vi "FRC Color Processing Example.vi"(8 "Image In":T1) -> ()   [LabVIEW 2015]
uses:
  <vilib>/vision/NI_Vision_Development_Module.lvlib
  Vision Support Code/Camera Types.ctl
  <vilib>/Rock Robotics/WPI/Camera/WPI_CameraSettings Read MJPG.ctl
  <vilib>/Rock Robotics/WPI/Camera/WPI_CameraImageSize.ctl
  <vilib>/vision/Image Controls.llb/IMAQ Image.ctl
panel:
  in  "Std Devs for Calibration":cluster{"H":dbl, "S":dbl, "V":dbl}={"H"=4.0, "S"=6.0, "V"=6.0}
  out "Highest Avg Score":dbl format="%#_3g"
  in  "Min Score Threshold":i32=70
  in  "Emphasize Limit Tests":bool=TRUE
  in  "Camera Type":T2=enum."MS HD3000 square"
  in  "image files":string[](array[string])
  in  "Aspect Ratio Fudge Factor":dbl=1.0
  out "Detected Targets":T3(array[cluster]) {"Normalized Rect"."Numeric 5" format="%#_2g"; "Normalized Rect"."Numeric 3" format="%#_2g"; "Normalized Rect"."Numeric 2" format="%#_2g"; "Normalized Rect"."Numeric" format="%#_2g"}
  in  "Annotation Limit":dbl=75.0
  in  "Source":enum32{"Files", "Camera"}(tab)
  in  "Images":i32(listbox)
  in  "Folder Location":path=path "C:/Program Files (x86)/National Instruments/LabVIEW 2015/examples/FRC/roboRIO/Vision/2016 Vision Example/Sample Images/Real Tower"
  in  "Camera Settings":T4={"fps"=20, "compression"=30, "Image Size"=enum."320x240"}
  in  "Camera Address":string="USB 1"
  in  "Annotate":bool=TRUE
  out "Sorted Particle Scores":T6(array[cluster]) {"Moment Factor" format="%#_3g"; "Aspect Ratio" format="%#_3g"; "Area to CH" format="%#_3g"; "X" format="%#_3g"; "Y" format="%#_3g"}
  out "Qualified Particles":i32
  in  "LED Color":T7={"Hue"={110.52399131877658, 148.6727294921875}, "Sat"={34.78571428571429, 255.0}, "Val"={91.07142857142858, 255.0}} {"Hue" scale=0.0..255.0 scale format="%#_3g"}
  out "Masked":T1(plugin-control)
  out "Original Image":T1(plugin-control)
  # "Instructions:\nUse Source to select image files from a directory, or use a USB or IP camera connected to your laptop.\nUse LED Color to threshold and build particles. Adjust HSV values to improve masking.\nClick and draw a line in Original Image to auto-calibrate to the LED color. You may need to widen Sat and Val.\nAnnotations draw a rectangle around \"good\" particles with scores from top to bottom."
  # "Density Profile"
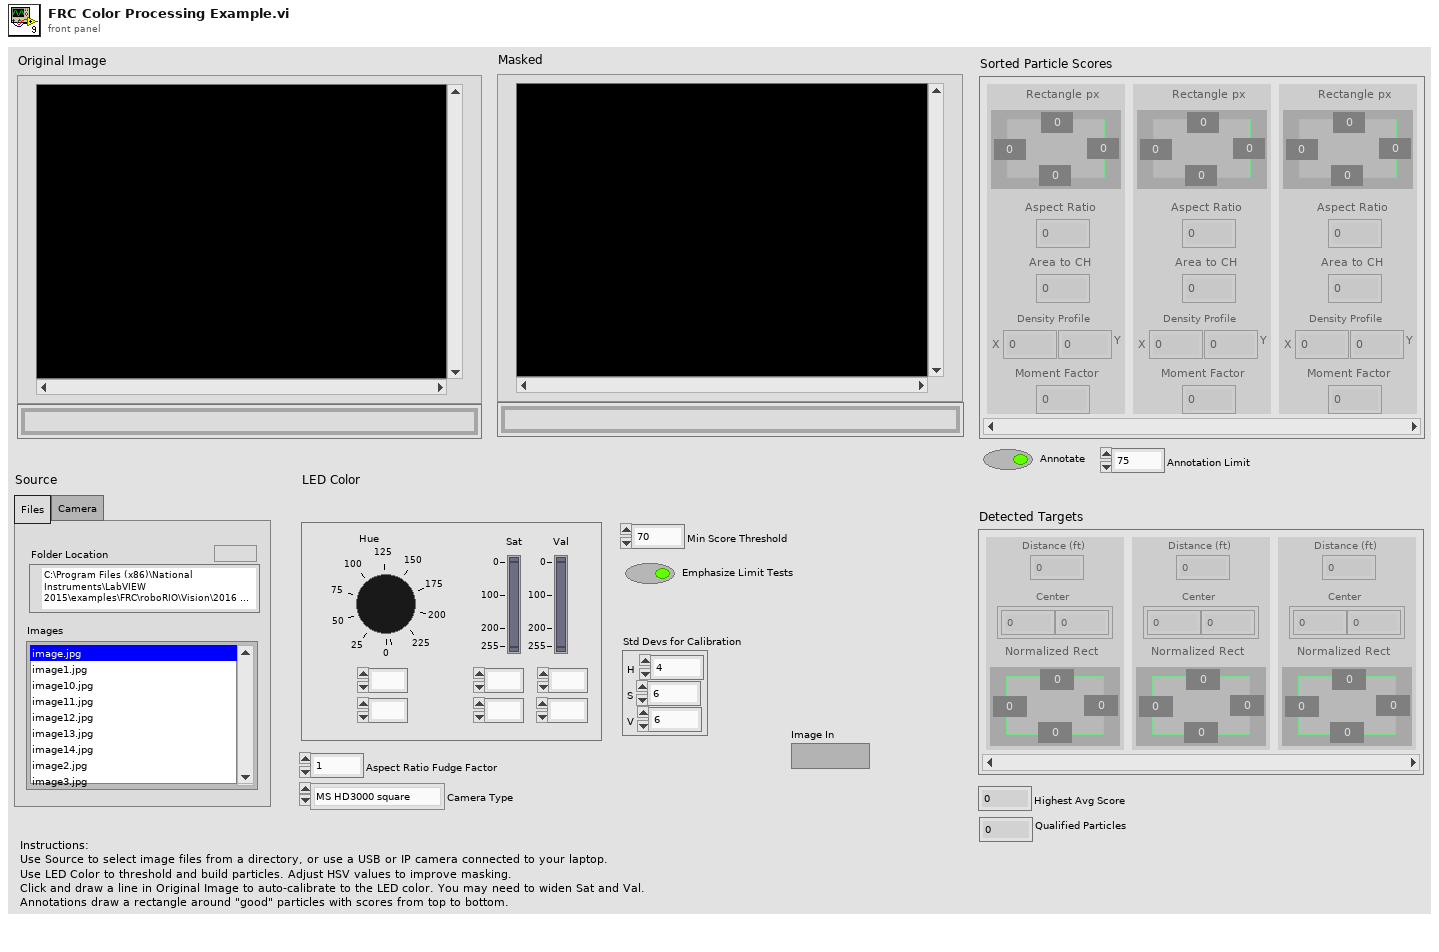
[diagram p1: front panel]
types:
  T1 = typedef "IMAQ Image.ctl" = refnum<image>
  T2 = typedef "Camera Types.ctl" = enum16{"206", "1011", "1013", "MS HD3000 square", "MS HD3000 640x480"}
  T3 = cluster{"Distance (ft)":dbl, "Center":cluster{dbl, dbl}, "Normalized Rect":cluster{"Numeric":dbl, "Numeric 2":dbl, "Numeric 3":dbl, "Numeric 5":dbl}}[]
  T4 = typedef "WPI_CameraSettings Read MJPG.ctl" = cluster{"fps":i32, "compression":i32, "Image Size":T5}
  T5 = typedef "WPI_CameraImageSize.ctl" = enum16{"640x480", "320x240", "160x120", "Custom"}
  T6 = cluster{"Rectangle px":cluster{"Numeric":dbl, "Numeric 2":dbl, "Numeric 3":dbl, "Numeric 5":dbl}, "Aspect Ratio":dbl, "Area to CH":dbl, "X":dbl, "Y":dbl, "Moment Factor":dbl}[]
  T7 = cluster{"Hue":cluster{dbl, dbl}, "Sat":cluster{dbl, dbl}, "Val":cluster{dbl, dbl}}
  T8 = typedef "Particle Parameters" = i32
  T9 = typedef "Image Type" = u32
  T10 = cluster{cluster{dbl, dbl}, cluster{dbl, dbl}, cluster{dbl, dbl}}
  T11 = cluster{"Bounding box":cluster{"left":dbl, "top":dbl, "right":dbl, "bottom":dbl}, "Aspect Ratio":dbl, "Area to CH":dbl, "X Mask":dbl, "Y Mask":dbl, "Moment":dbl}[]
  T12 = cluster{"Rectangle":cluster{"Numeric":dbl, "Numeric 2":dbl, "Numeric 3":dbl, "Numeric 5":dbl}, "L":dbl, "Area to CH":dbl, "X":dbl, "Y":dbl, "Moment Factor":dbl}[]
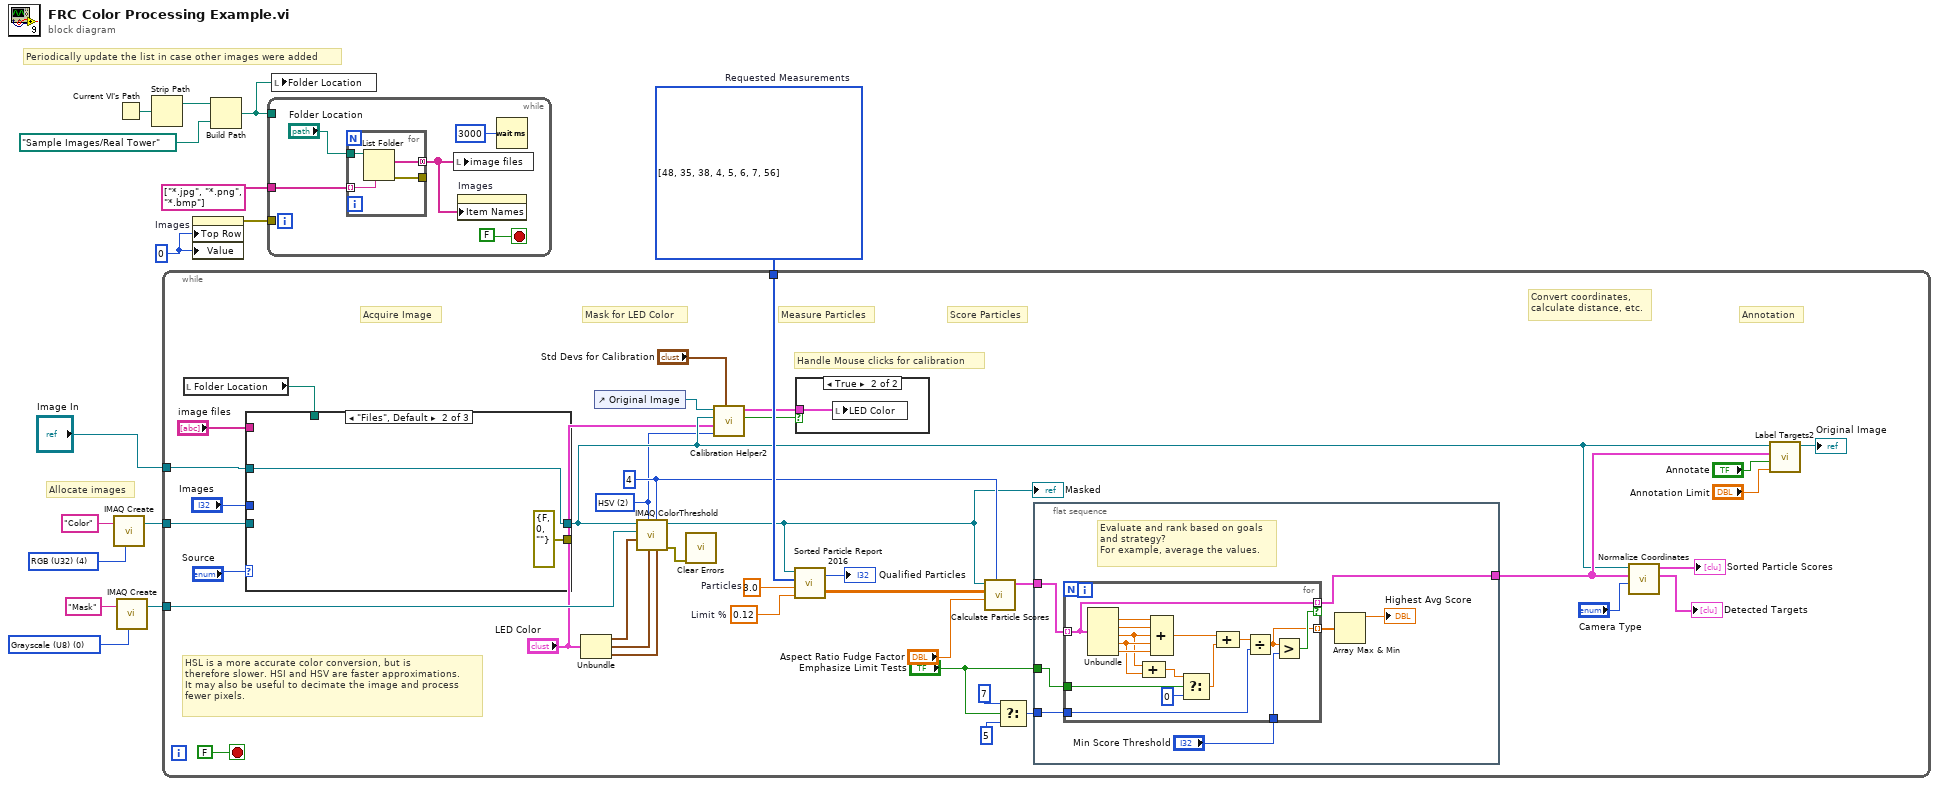
[diagram p0: block diagram]
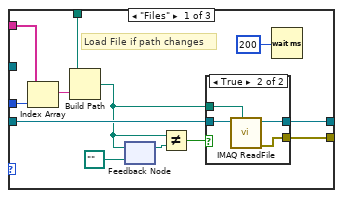
[diagram p3: hidden frame]
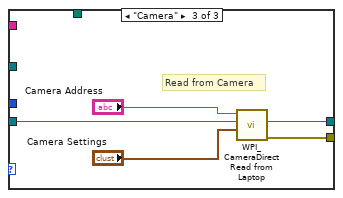
[diagram p5: hidden frame]
diagram:
  w3 = u32 0 ("milliseconds to wait")
  w9 = T8[] [48, 35, 38, 4, 5, 6, 7, 56] items=["Center of Mass X", "Center of Mass Y", "First Pixel X", "First Pixel Y", "Bounding Rect Left", "Bounding Rect Top", "Bounding Rect Right", "Bounding Rect Bottom", "Max Feret Diameter Start X", "Max Feret Diameter Start Y", "Max Feret Diameter End X", "Max Feret Diameter End Y", "Max Horiz. Segment Length Left", "Max Horiz. Segment Length Right", "Max Horiz. Segment Length Row", "-", "Bounding Rect Width", "Bounding Rect Height", "Bounding Rect Diagonal", "Perimeter", "Convex Hull Perimeter", "Holes' Perimeter", "Max Feret Diameter", "Equivalent Ellipse Major Axis", "Equivalent Ellipse Minor Axis", "Equivalent Ellipse Minor Axis (Feret)", "Equivalent Rect Long Side", "Equivalent Rect Short Side", "Equivalent Rect Diagonal", "Equivalent Rect Short Side (Feret)", "Average Horiz. Segment Length", "Average Vert. Segment Length", "Hydraulic Radius", "Waddel Disk Diameter", "-", "Area", "Holes' Area", "Particle & Holes' Area", "Convex Hull Area", "Image Area", "-", "Number of Holes", "Number of Horiz. Segments", "Number of Vert. Segments", "-", "Orientation", "Max Feret Diameter Orientation", "-", "% Area/Image Area", "% Area/(Particle & Holes' Area)", "Ratio of Equivalent Ellipse Axes", "Ratio of Equivalent Rect Sides", "-", "Elongation Factor", "Compactness Factor", "Heywood Circularity Factor", "Type Factor", "-", "Sum X", "Sum Y", "Sum XX", "Sum XY", "Sum YY", "Sum XXX", "Sum XXY", "Sum XYY", "Sum YYY", "-", "Moment of Inertia XX", "Moment of Inertia XY", "Moment of Inertia YY", "Moment of Inertia XXX", "Moment of Inertia XXY", "Moment of Inertia XYY", "Moment of Inertia YYY", "Norm. Moment of Inertia XX", "Norm. Moment of Inertia XY", "Norm. Moment of Inertia YY", "Norm. Moment of Inertia XXX", "Norm. Moment of Inertia XXY", "Norm. Moment of Inertia XYY", "Norm. Moment of Inertia YYY", "Hu Moment 1", "Hu Moment 2", "Hu Moment 3", "Hu Moment 4", "Hu Moment 5", "Hu Moment 6", "Hu Moment 7"]  # Requested Measurements
  w12 = T9 0 items=["Grayscale (U8)", "Grayscale (I16)", "Grayscale (SGL)", "Complex (CSG)", "RGB (U32)", "HSL (U32)", "RGB (U64)", "Grayscale (U16)"] ("Image Type")
  w14 = T9 4 items=["Grayscale (U8)", "Grayscale (I16)", "Grayscale (SGL)", "Complex (CSG)", "RGB (U32)", "HSL (U32)", "RGB (U64)", "Grayscale (U16)"] ("Image Type")
  # "Periodically update the list in case other images were added"
  # "Allocate images"
  n1 = call "IMAQ Create"("Image Name"="Color", "Image Type"=w14) -> ("New Image"=w13:T1)  [unwired: 2 in, 2 out]
  n2 = Current VI's Path() -> (path=w8:path)
  n3 = call "IMAQ Create"("Image Name"="Mask", "Image Type"=w12) -> ("New Image"=w10:T1)  [unwired: 2 in, 2 out]
  n4 = Strip Path(path=w8) -> (stripped path=w6:path)  [unwired: 1 out]
  n5 = while {
    tunnel: w13 -> [w53]
    tunnel: w10 -> [w51]
    tunnel: w9 -> [w47]
    tunnel: "Image In" -> [w16]
    stop <- FALSE stop-if-true
    w39 = 4 ("Replace Value")
    w43 = 0.12  # Limit %
    w46 = 3.0  # Particles
    w21 = u16 2 items=["RGB", "HSL", "HSV", "HSI"] ("Color Mode")
    # "Handle Mouse clicks for calibration"
    # "Measure Particles"
    # "Convert coordinates,\ncalculate distance, etc."
    # "Annotation"
    # "Score Particles"
    # "Mask for LED Color"
    # "Acquire Image"
    # "HSL is a more accurate color conversion, but is\ntherefore slower. HSI and HSV are faster approximations.\nIt may also be useful to decimate the image and process\nfewer pixels."
    n6 = local read "Folder Location"() -> (w18:path)
    n7 = case shown="Default, \"Robot\"" "Source" {
      tunnel: [w89 errorcluster {"status"=FALSE, "code"=0, "source"=""} ("error out") w102] -> _
      tunnel: [w90 w97 w101] -> w24
      tunnel: w53 -> [w88 _ w100]
      tunnel: "image files" -> [w80 _ _]
      tunnel: "Images" -> [w87 _ _]
      tunnel: w18 -> [w85 _ _]
      tunnel: w16 -> [_ w97 _]
      frame "Files" {
        # "Load File if path changes"
        n8 = Index Array(array=w80, index=w87) -> (element=w86:string)
        n9 = Build Path(base path=w85, name or relative path=w86) -> (appended path=w81:path)
        n10 = feedback-in #1(w81) -> ()
        n11 = feedback #1(path "" ("appended path")) -> (w83:path)
        n12 = Not Equal?(x=w81, y=w83) -> (x != y?=w84:bool)
        n13 = case shown="True" w84 {
          tunnel: [w91 w95] -> w90
          tunnel: [_ w94] -> w89
          tunnel: w88 -> [w91 w93]
          tunnel: w81 -> [_ w92]
          frame False {
          }
          frame True {
            n14 = call "IMAQ ReadFile"("File Path"=w92, "Image"=w93) -> ("error out"=w94:errorcluster, "Image Out"=w95:T1)  [unwired: 5 in, 3 out]
          }
        }
        n15 = Wait (ms)(milliseconds to wait=u32 200 ("delay (ms)")) -> ()  [unwired: 1 out]
      }
      frame "Files", Default {
      }
      frame "Camera" {
        # "Read from Camera"
        n16 = call <vilib>:"WPI_CameraDirect Read from Laptop.vi"("Camera Settings"="Camera Settings", "Image"=w100, "address"="Camera Address") -> ("error out"=w102:errorcluster, "Image Out"=w101:T1)  [unwired: 7 in]
      }
    }
    n17 = Unbundle("LED Color") -> ("Hue"=w50:cluster{dbl, dbl}, "Sat"=w49:cluster{dbl, dbl}, "Val"=w48:cluster{dbl, dbl})
    n18 = control-ref of="Original Image"() -> (w25:refnum<vi>)
    n19 = call "IMAQ ColorThreshold"("Blue or Luma or Val or Inten Range"=w48, "Replace Value"=w39, "Green or Sat Range"=w49, "Color Mode"=w21, "Red or Hue Range"=w50, "Image Dst"=w51, "Image Src"=w24) -> ("error out"=w29:errorcluster, "Image Dst Out"=w30:T1)  [unwired: 3 in]
    "Masked" <- w30
    n20 = call <vilib>:"Clear Errors.vi"("error in (no error)"=w29) -> ()  [unwired: 5 in, 2 out]
    n21 = call "Calibration Helper2.vi"("Std Devs"="Std Devs for Calibration", "Color Mode"=w21, "Color Components"="LED Color", "Image"=w24, "Image Ctl Refnum"=w25) -> ("Changed"=w23:bool, "output color"=w22:T10)  [unwired: 5 in]
    n22 = call "Sorted Particle Report 2016.vi"("Min Area Size %"=w43, "Particle Count Limit"=w46, "Pixel Measurements"=w47, "Image in"=w30) -> ("Sorted Data"=w44:dbl[][], "Particles"=→"Qualified Particles":i32)
    n23 = case shown="True" w23 {
      tunnel: w22 -> [_ w55]
      frame False {
      }
      frame True {
        n24 = local write "LED Color"(w55) -> ()
      }
    }
    n25 = call "Calculate Particle Scores.vi"("Pixel Value"=w39, "Aspect Fudge Factor"="Aspect Ratio Fudge Factor", "Sorted Data"=w44, "Image in"=w30) -> ("Scores"=w33:T11)  [unwired: 7 in]
    n26 = Select(t=7, s="Emphasize Limit Tests", f=5) -> (s? t:f=w26:i32)
    n27 = flat-sequence {
      tunnel: w33 -> [w61]
      tunnel: [w62] -> w31
      tunnel: w26 -> [w58]
      tunnel: "Emphasize Limit Tests" -> [w56]
      frame #0 {
        # "Evaluate and rank based on goals\nand strategy?\nFor example, average the values."
        n28 = for {
          tunnel: w61 -> [w76] mode=indexing
          tunnel: [w76] -> w62 mode=indexing if=w75
          tunnel: [w74] -> w60 mode=indexing
          tunnel: w58 -> [w73]
          tunnel: "Min Score Threshold" -> [w72]
          tunnel: w56 -> [w65]
          n29 = Unbundle(w76) -> ("Aspect Ratio"=w78:dbl, "Area to CH"=w77:dbl, "X Mask"=w67:dbl, "Y Mask"=w68:dbl, "Moment"=w69:dbl)  [unwired: 1 out]
          n30 = Compound Arithmetic op=ADD(w67, w68) -> (w66:dbl)
          n31 = Compound Arithmetic op=ADD(w78, w77, w67, w68, w69) -> (w71:dbl)
          n32 = Select(t=w66, s=w65, f=0) -> (s? t:f=w64:dbl)
          n33 = Compound Arithmetic op=ADD(w71, w64) -> (w70:dbl)
          n34 = Divide(x=w70, y=w73) -> (x/y=w74:dbl)
          n35 = Greater?(x=w74, y=w72) -> (0:w75:bool)
        }
        n36 = Array Max & Min(array=w60) -> (max value=→"Highest Avg Score":dbl)  [unwired: 3 out]
      }
    }
    n37 = call "Normalize Coordinates.vi"("Camera Type"="Camera Type", "Targets"=w31, "Image in"=w24) -> ("Found Targets"=→"Detected Targets":T3, "Sorted Scores"=→"Sorted Particle Scores":T12)  [unwired: 7 in]
    n38 = call "Label Targets2.vi"("Score Threshold"="Annotation Limit", "Annotate"="Annotate", "Targets"=w31, "Image in"=w24) -> ("Image out"=→"Original Image":T1)  [unwired: 7 in]
  }
  n39 = property on="Images" class="LstBox (strict)"("Top Row"=w3, "Value"=w3) -> (error out=w4:errorcluster)  [unwired: 2 in, 1 out]
  n40 = Build Path(base path=w6, name or relative path=path "Sample Images/Real Tower" ("Folder Location")) -> (appended path=w5:path)
  n41 = while {
    tunnel: w5 -> [_]
    tunnel: w4 -> [_]
    tunnel: string[] ["*.jpg", "*.png", "*.bmp"] -> [w103]
    stop <- FALSE stop-if-true
    n42 = for {
      tunnel: [w111] -> w105 mode=concatenating
      tunnel: "Folder Location" -> [w110]
      tunnel: [w109] -> _
      tunnel: w103 -> [w108] mode=indexing
      n43 = List Folder(path=w110, pattern=w108) -> (filenames=w111:string[], error out=w109:errorcluster)  [unwired: 2 in, 2 out]
    }
    n44 = local write "image files"(w105) -> ()
    n45 = property on="Images" class="LstBox (strict)"("Item Names"=w105) -> ()  [unwired: 2 in, 2 out]
    n46 = Wait (ms)(milliseconds to wait=u32 3000) -> ()  [unwired: 1 out]
  }
  n47 = local write "Folder Location"(w5) -> ()
